vi "Send Next.vi"(7 "command":T1=enum."Rx", 8 "error in (no error)":errorcluster, 9 "Plugin ID":i32, 10 "Dispatcher Interface":refnum<class "Dispatcher Interface.lvclass">, 11 "Transfer Group in":refnum<class "Transfer Group.lvclass">) -> (0 "error out":errorcluster, 3 "Transfer Group out":refnum<class "Transfer Group.lvclass">)   [LabVIEW 2017, in "DSF Core.lvlib" / "Transfer Group.lvclass"]
uses:
  Transfer Group.lvclass
  Interface/Dispatcher/Dispatcher Interface.lvclass
  Interface/Dispatcher/Command.ctl
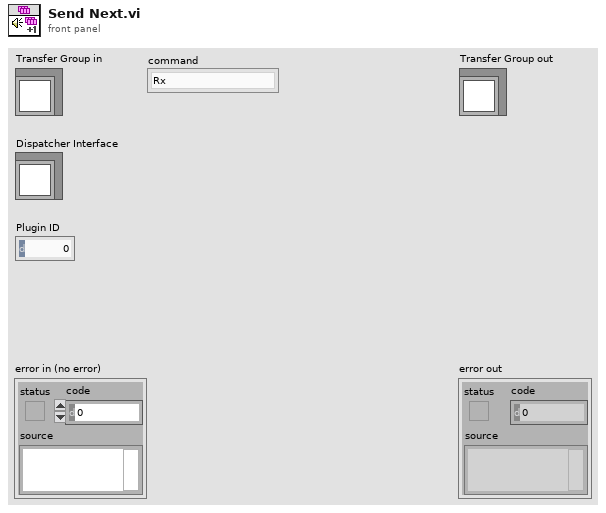
[diagram p1: front panel]
types:
  T1 = typedef "DSF Core.lvlib/Dispatcher Interface.lvclass/Command.ctl" = enum8{"Idle", "Start", "Rx", "Tx", "Set Inline Buffer", "Shutdown", "Error"}
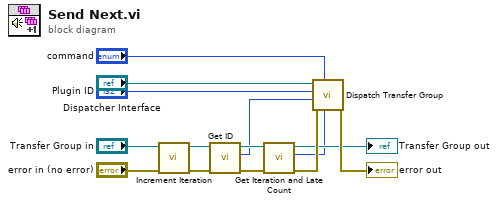
[diagram p0: block diagram]
diagram:
  n1 = call "Increment Iteration.vi"("error in (no error)"="error in (no error)", "Transfer Group in"="Transfer Group in") -> ("error out"=w11:errorcluster, "Transfer Group out"=w13:refnum<class "Transfer Group.lvclass">)  [unwired: 8 in]
  n2 = call "Get ID.vi"("Transfer Group in"=w13) -> ("id"=w10:i32, "Transfer Group out"=w12:refnum<class "Transfer Group.lvclass">)  [unwired: 9 in]
  n3 = call "Get Iteration and Late Count.vi"("error in (no error)"=w11, "Transfer Group in"=w12) -> ("error out"=w9:errorcluster, "iteration"=w3:u64, "Transfer Group out"=→"Transfer Group out":refnum<class "Transfer Group.lvclass">)  [unwired: 6 in, 1 out]
  n4 = call "Dispatch Transfer Group.vi"("Iteration"=w3, "command"="command", "error in (no error)"=w9, "Transfer Group ID"=w10, "Plugin ID"="Plugin ID", "Dispatcher Interface in"="Dispatcher Interface") -> ("error out"=→"error out":errorcluster)  [unwired: 4 in, 1 out]
